vi "A33ConfigureBurst.vi"(1 "Internal period":sgl=0.1 format="%_12g", 4 "Burst phase (-360..+360)":sgl format="%_12g", 5 "Gate polarity (F: positive)":bool, 6 "Burst Count (1-100M)":i32=1, 7 "Enable Burst (T: Enable)":bool=TRUE, 8 "error in (no error)":errorcluster, 9 "Burst Mode (0: Triggered)":u16(ring) items=["Triggered", "Gated"], 10 "Channel (0: Channel 1)":u16(ring) items=["Channel 1"=1, "Channel 2"=2], 11 "VISA resource name":refnum<visa-resource-name>) -> (0 "error out":errorcluster, 3 "VISA resource name out":refnum<visa-resource-name>)   [LabVIEW 2022 SP3]
doc: "Allows and configures burst modulation. Configures the function generator to output a waveform with specified number of cycles, called burst. The carrier waveform shape and parameters are set by Configure Standard Waveform."
panel:
  # "Phase is not delay!!"
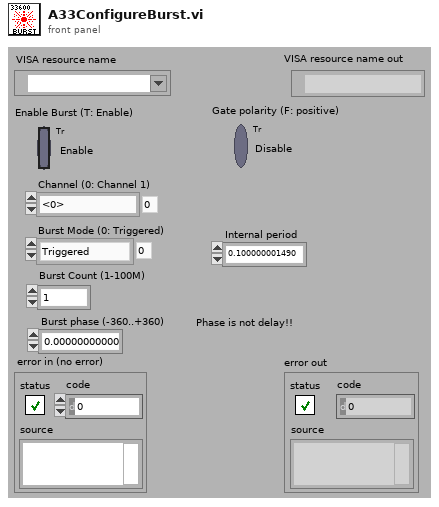
[diagram p1: front panel]
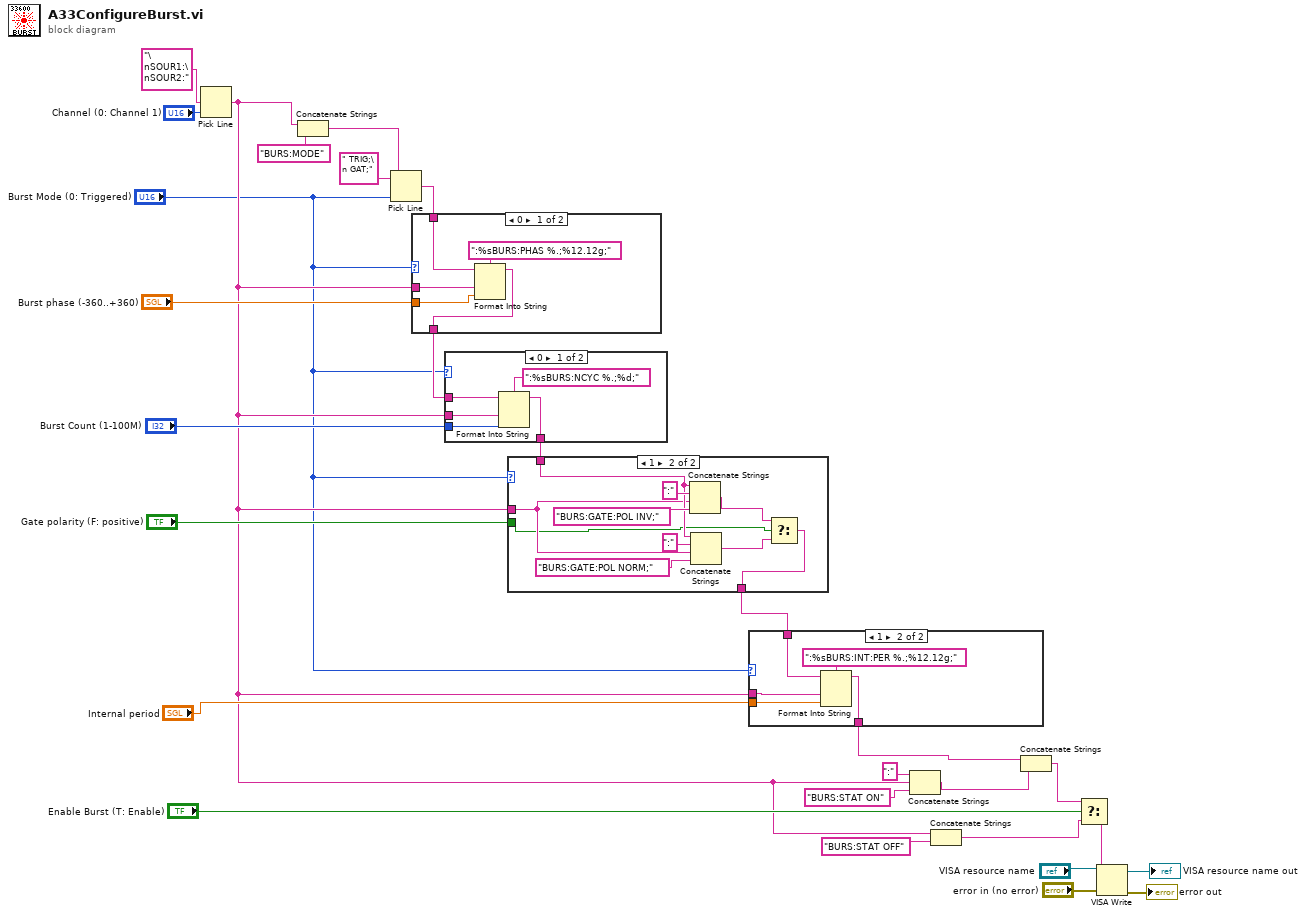
[diagram p0: block diagram]
diagram:
  n1 = Pick Line(multi-line string="\nSOUR1:\nSOUR2:" ("string (\"\")"), line index="Channel (0: Channel 1)") -> (output string=w4:string)  [unwired: 1 in]
  n2 = Concatenate Strings(w4, "BURS:MODE" ("format string")) -> (w20:string)
  n3 = Pick Line(string ("")=w20, multi-line string=" TRIG;\n GAT;" ("string (\"\")"), line index="Burst Mode (0: Triggered)") -> (output string=w17:string)
  n4 = case shown="0" "Burst Mode (0: Triggered)" {
    tunnel: w17 -> [w32 w34]
    tunnel: [w29 w34] -> w16
    tunnel: w4 -> [w31 _]
    tunnel: "Burst phase (-360..+360)" -> [w30 _]
    frame 0 {
      n5 = Format Into String(format string=":%sBURS:PHAS %.;%12.12g;", initial string=w32, w31, w30) -> (resulting string=w29:string)  [unwired: 1 in, 1 out]
    }
    frame 1, Default {
    }
  }
  n6 = case shown="0" "Burst Mode (0: Triggered)" {
    tunnel: [w38 w40] -> w7
    tunnel: "Burst Count (1-100M)" -> [w37 _]
    tunnel: w16 -> [w36 w40]
    tunnel: w4 -> [w35 _]
    frame 0 {
      n7 = Format Into String(format string=":%sBURS:NCYC %.;%d;", initial string=w36, w35, w37) -> (resulting string=w38:string)  [unwired: 1 in, 1 out]
    }
    frame 1, Default {
    }
  }
  n8 = case shown="1" "Burst Mode (0: Triggered)" {
    tunnel: w7 -> [w41 w45]
    tunnel: w4 -> [_ w44]
    tunnel: [w41 w43] -> w2
    tunnel: "Gate polarity (F: positive)" -> [_ w42]
    frame 0, Default {
    }
    frame 1 {
      n9 = Concatenate Strings(w45, ":" ("string"), w44, "BURS:GATE:POL INV;" ("string")) -> (w48:string)
      n10 = Concatenate Strings(w45, ":" ("string"), w44, "BURS:GATE:POL NORM;" ("string")) -> (w51:string)
      n11 = Select(t=w48, s=w42, f=w51) -> (s? t:f=w43:string)
    }
  }
  n12 = case shown="1" "Burst Mode (0: Triggered)" {
    tunnel: "Internal period" -> [_ w56]
    tunnel: w4 -> [_ w55]
    tunnel: [w52 w54] -> w3
    tunnel: w2 -> [w52 w53]
    frame 0, Default {
    }
    frame 1 {
      n13 = Format Into String(format string=":%sBURS:INT:PER %.;%12.12g;", initial string=w53, w55, w56) -> (resulting string=w54:string)  [unwired: 1 in, 1 out]
    }
  }
  n14 = Concatenate Strings(":" ("string"), w4, "BURS:STAT ON" ("string")) -> (w9:string)
  n15 = Concatenate Strings(w4, "BURS:STAT OFF" ("string")) -> (w19:string)
  n16 = Concatenate Strings(w3, w9) -> (w25:string)
  n17 = Select(t=w25, s="Enable Burst (T: Enable)", f=w19) -> (s? t:f=w24:string)
  n18 = VISA Write(VISA resource name="VISA resource name", write buffer=w24, error in (no error)="error in (no error)") -> (VISA resource name out=→"VISA resource name out":refnum<visa-resource-name>, error out=→"error out":errorcluster)  [unwired: 1 out]
